vi "Close.vi"(0 "Manual Cal Standard in":refnum<class "Cal Standard.lvclass">, 11 "error in (no error)":errorcluster) -> (4 "Manual Cal Standard out":refnum<class "Cal Standard.lvclass">, 15 "error out":errorcluster)   [LabVIEW 2023, in "Manual Cal Standard.lvlib" / "Cal Standard.lvclass"]
uses:
  Cal Standard.lvclass
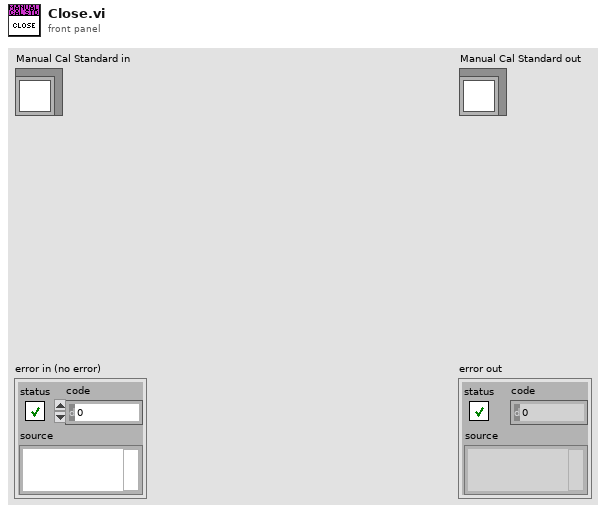
[diagram p1: front panel]
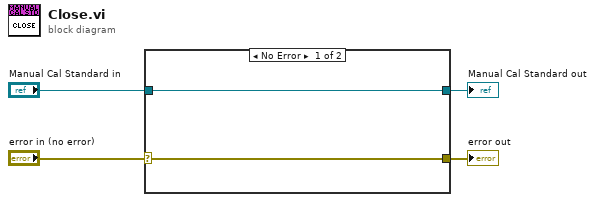
[diagram p0: block diagram]
diagram:
  n1 = case shown="No Error" "error in (no error)" {
    selector: "error in (no error)" -> [w5 w8]
    tunnel: [w5 w8] -> w1
    tunnel: [w6 w7] -> w3
    tunnel: "Manual Cal Standard in" -> [w6 w7]
    frame No Error {
    }
    frame Error {
    }
  }
  "error out" <- w1
  "Manual Cal Standard out" <- w3
